vi "Set Comm Timeout Val V.vi"(8 "error in (no error)":errorcluster, 10 "WriteTimeout":i16, 11 "ReadTimeout":i16) -> (0 "error out":errorcluster, 3 "function return":i16)   [LabVIEW 2009, in "VantagePro.lvlib"]
doc: "DllAccess short int _stdcall SetCommTimeoutVal_V(short int ReadTimeout, short int WriteTimeout);"
uses:
  VantagePro.lvlib
  <userlib>/VantagePro/VantagePro.dll
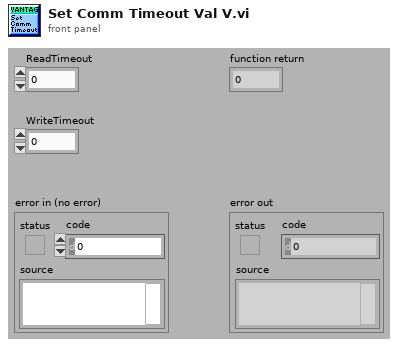
[diagram p1: front panel]
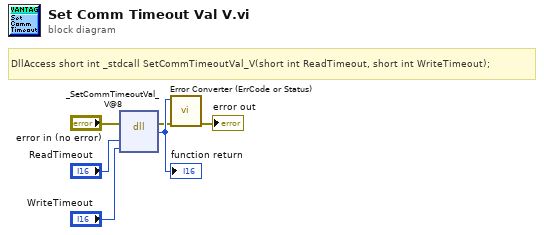
[diagram p0: block diagram]
diagram:
  # "DllAccess short int _stdcall SetCommTimeoutVal_V(short int ReadTimeout, short int WriteTimeout);"
  n1 = dll-call lib="C:/Program Files/National Instruments/LabVIEW 2010/user.lib/VantagePro/VantagePro.*" fn="_SetCommTimeoutVal_V@8"(error in="error in (no error)", "ReadTimeout"="ReadTimeout", "WriteTimeout"="WriteTimeout") -> (error out=w2:errorcluster, w6:i16)  [unwired: 4 in, 1 out]
  "function return" <- w6
  n2 = call "Error Converter (ErrCode or Status).vi"("error in (no error)"=w2, "error code"=w6) -> ("error out"=→"error out":errorcluster)  [unwired: 9 in]
